vi "SRV_XModem_GetPacket.vi"(2 "text":string, 3 "X reply":string, 4 "packet #":i32) -> (1 "Block":T1 {"Complement" format="%.0x"; "Packet Number" format="%.0x"})   [LabVIEW 2014]
doc: "Modified: Mike Schultz - Logic PD"
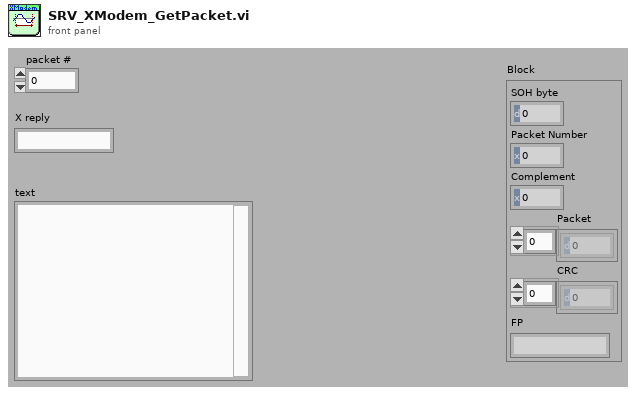
[diagram p1: front panel]
types:
  T1 = cluster{"SOH byte":u8, "Packet Number":u8, "Complement":u8, "Packet":u8[], "CRC":u8[], "FP":string}
  T2 = cluster{"SOH":u8, u8, u8, u8[], "CRC":u8[], "string":string}
  T3 = cluster{"SOH":u8, u8, u8, u8[], "16-bit CRC Array":u8[], "string":string}
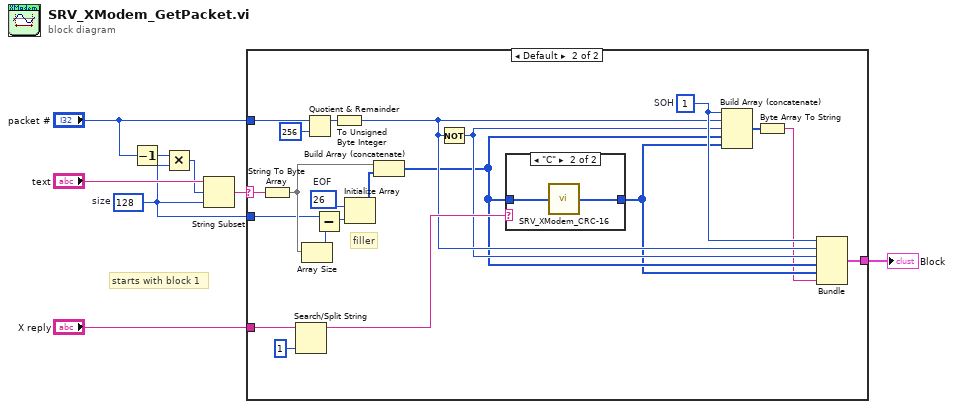
[diagram p0: block diagram]
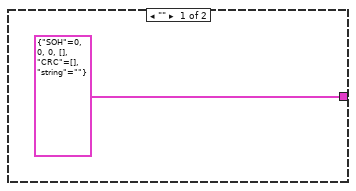
[diagram p2: hidden frame]
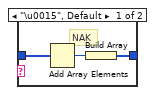
[diagram p3: hidden frame]
diagram:
  w2 = u8 128  # size
  # "starts with block 1"
  n1 = Decrement(x="packet #") -> (x-1=w1:i32)
  n2 = Multiply(x=w1, y=w2) -> (x*y=w6:i32)
  n3 = String Subset(string="text", offset (0)=w6, length (rest)=w2) -> (substring=w5:string)
  n4 = case shown="Default" w5 {
    selector: w5 -> [_ w22]
    tunnel: [T2 {"SOH"=0, 0, 0, [], "CRC"=[], "string"=""} w30] -> w7
    tunnel: "X reply" -> [_ w20]
    tunnel: w2 -> [_ w23]
    tunnel: "packet #" -> [_ w17]
    frame "" {
    }
    frame Default {
      w27 = u8 26  # EOF
      w15 = u8 1  # SOH
      # "filler"
      n5 = String To Byte Array(string=w22) -> (unsigned byte array=w25:u8[])
      n6 = Search/Split String(string=w20, offset (0)=1) -> (substring before match=w19:string)  [unwired: 1 in, 2 out]
      n7 = Array Size(array=w25) -> (size(s)=w28:i32)
      n8 = Quotient & Remainder(x=w17, y=u32 256) -> (x-y*floor(x/y)=w16:u32)  [unwired: 1 out]
      n9 = Subtract(x=w23, y=w28) -> (x-y=w26:i32)
      n10 = To Unsigned Byte Integer(number=w16) -> (unsigned 8bit integer=w14:u8)
      n11 = Initialize Array(w27, w26) -> (w24:u8[])
      n12 = Build Array (concatenate)(w25, w24) -> (w12:u8[])
      n13 = Not(x=w14) -> (.not. x?=w13:u8)
      n14 = case shown="\"C\"" w19 {
        tunnel: w12 -> [w32 w35]
        tunnel: [w31 w34] -> w11
        frame "\u0015", Default {
          # "NAK"
          n15 = Add Array Elements(numeric array=w32) -> (sum=w33:u8)
          n16 = Build Array(w33) -> (w31:u8[])
        }
        frame "C" {
          n17 = call "SRV_XModem_CRC-16.vi"("Array"=w35) -> ("16-bit CRC Array"=w34:u8[])  [unwired: 14 in]
        }
      }
      n18 = Build Array (concatenate)(w15, w14, w13, w12, w11) -> (w29:u8[])
      n19 = Byte Array To String(unsigned byte array=w29) -> (string=w10:string)
      n20 = Bundle("SOH"=w15, w14, w13, w12, "16-bit CRC Array"=w11, "string"=w10) -> (w30:T3)  [unwired: 1 in]
    }
  }
  "Block" <- w7
